vi "Set laser power.vi"(8 "error in (no error)":errorcluster, 11 "Laser power %":u8) -> (0 "error out":errorcluster)   [LabVIEW 2017]
uses:
  Global Variables/gl_UI Ctrl Refs.vi
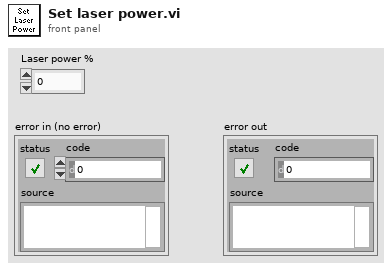
[diagram p1: front panel]
types:
  T1 = typedef "UI ctrl refs cluster.ctl" = cluster{"Top level VI path":path, "Top level VI ref":refnum<vi>, "User menu ref":refnum<k9>, "Sub Panel control":refnum<vi>, "Imaging Param Tab":refnum<vi>, "Occurrence-Start drivers":refnum<k4>, "Occurrence-Speed logging initialised":refnum<k4>, "Occurrence-XYZ stage initialised":refnum<k4>, "Exit button":refnum<vi>, "Status ind":refnum<vi>, "Set as origin":refnum<vi>, "Speed Logging":refnum<vi>, "Time Lapse":refnum<vi>, "Live Imaging":refnum<vi>, "AOL Z Stack":refnum<vi>, "Motor Z Stack":refnum<vi>, "Funct Acq button":refnum<vi>, "Hard Shutter":refnum<vi>, "Virtual Shutter":refnum<vi>, "Laser Power":refnum<vi>, "AOL Mode":refnum<vi>, "Frame Size":refnum<vi>, "Field of View":refnum<vi>, "Dwell Time":refnum<vi>, "Zoom":refnum<vi>, "AOL Z":refnum<vi>, "Objective":refnum<vi>, "Axis":refnum<vi>, "Paths & Names":refnum<vi>, "Experiment folder path (ind.)":refnum<vi>, "Last State (Ind.)":refnum<vi>, "Laser wavelength ind (nm)":refnum<vi>, "Averages":refnum<vi>, "Angle (degrees)":refnum<vi>, "X centre":refnum<vi>, "Y centre":refnum<vi>, "Plane Mode":refnum<vi>, "# Planes":refnum<vi>, "Z Start":refnum<vi>, "Z Stop":refnum<vi>, "Z Step":refnum<vi>, "PMT 1":refnum<vi>, "PMT 2":refnum<vi>, "Stage XYZ Position":refnum<vi>, "Pockels@Z Start":refnum<vi>, "Pockels@Z Stop":refnum<vi>, "Obtain Z Start":refnum<vi>, "Obtain Z Stop":refnum<vi>, "Live stim.trig.period":refnum<vi>, "Live stim.trig.enable":refnum<vi>, "Movement Correction":refnum<vi>, "Load Reference Image":refnum<vi>, "XY Stage Move":refnum<vi>, "MovCor Cluster":refnum<vi>, "RefDAQParam":refnum<vi>, "Funct. Acq. Pockels Modulation":refnum<vi>, "Background MovCor":refnum<vi>, "Ref Laser Power":refnum<vi>, "Enable Video Recording":refnum<vi>, "Video Record-Live Imaging":refnum<vi>, "Video Record-Funct acq":refnum<vi>, "Reference Source":refnum<vi>, "AOL Z-stack Chirps Ready (ind)":refnum<vi>, "Target time between mov.cor. ref triggers (ms)":refnum<vi>, "Funct. Acq. Ref frame save":refnum<vi>, "Tracking button":refnum<vi>, "Show ref plots window":refnum<vi>, "Center freq ind (nm)":refnum<vi>, "Pickup mode (ind)":refnum<vi>, "Logging queue (ind)":refnum<vi>, "Back aperture power (ind.)":refnum<vi>, "Power after objective (ind.)":refnum<vi>, "Switch user":refnum<vi>}
  T2 = typedef "AOL_Globals.ctl" = cluster{"Imaging Protocol":T3, "Number of POI":u16, "Number of Miniscans":u16, "Number of Trials":u16, "Number of Cycles ":u64, "# Averaged Frames":u16, "Laser power (%)":u8, "Pockels":dbl, "Acquisition Length (sec)":dbl, "Fill time (us)":dbl, "POI Dwell time (us)":dbl, "Miniscan Dwell time per pixel (us)":dbl, "PMT 1":dbl, "PMT 2":dbl, "Back Apperture":dbl, "Frame Size":T4, "Center Frequency":dbl, "Field of View":dbl, "DwellTime (us)":dbl, "Wavelength (nm)":dbl, "Zoom":dbl, "AOL Z":dbl, "AOL Mode":T5, "GridXY":dbl, "GridZ":dbl, "TriggerPeriod (sec)":dbl, "Number of Pixels in Miniscan":u16, "Experiment folder path":path, "X centre":dbl, "Y centre":dbl, "Angle (degrees)":dbl, "Plane Mode":T6, "Threshold":u16[], "Regenerate Chirps":bool, "Rectangle ROI length (pixels)":u16, "Rectangle ROI height (pixels)":u16, "AOD fill":u16, "StartupDelay":i32, "Samples Wait after Trigger":u16, "Slip Cycle":u32, "Add Cycle":bool}
  T3 = typedef "Imaging Protocols enum.ctl" = enum16{"AOL Z-Stack", "Motor Z Stack", "Functional Acquisition", "Single Plane Acquisition", "Volume Acquisition", "Live Imaging", "Live Plane Imaging", "Live Volume Imaging"}
  T4 = typedef "Frame Size.ctl" = u16
  T5 = typedef "AOL modes.ctl" = enum16{"Raster", "Structural", "Pointing", "Mini Scan", "Alignment"}
  T6 = typedef "Plane Mode.ctl" = u16
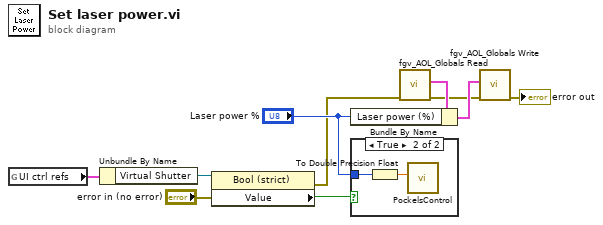
[diagram p0: block diagram]
diagram:
  n1 = global read "gl_UI Ctrl Refs.vi" "UI ctrl refs"() -> (w6:T1)
  n2 = Unbundle By Name(w6) -> ("Virtual Shutter"=w5:refnum<vi>)
  n3 = property class="Bool (strict)"(reference=w5, error in="error in (no error)") -> (error out=w2:errorcluster, "Value"=w9:bool)  [unwired: 1 out]
  n4 = case shown="True" w9 {
    tunnel: "Laser power %" -> [_ w12]
    frame False {
    }
    frame True {
      n5 = To Double Precision Float(number=w12) -> (double precision float=w11:dbl)
      n6 = call "PockelsControl.vi"("Laser Power (%)"=w11) -> ()  [unwired: 10 in, 1 out]
    }
  }
  n7 = call "fgv_AOL_Globals Read.vi"("error in (no error)"=w2) -> ("error out"=w4:errorcluster, "AOL_Globals"=w8:T2)  [unwired: 8 in, 1 out]
  n8 = Bundle By Name(cluster=w8, "Laser power (%)"="Laser power %") -> (w7:T2)
  n9 = call "fgv_AOL_Globals Write.vi"("error in (no error)"=w4, "AOL_Globals"=w7) -> ("error out"=→"error out":errorcluster)  [unwired: 9 in]
